vi "S2DS_Open dstp for external write (SubVI).vi"(8 "error in (no error)":errorcluster, 9 "Number identifier":i32, 10 "External Write instrument settings":T2={"Check for response?"=FALSE, "Pooling time out (ms)"=0, "Precision"=0.0, "IP"="localhost"}, 11 "Instrument parameters in":T1) -> (0 "error out":errorcluster, 1 "Read port list":string[](array[string]), 2 "Write port list":string[](array[string]), 3 "Instrument parameters out":T1)   [LabVIEW 2025]
uses:
  TYPE DEFS/S2DS_External write instrument settings.ctl
  TYPE DEFS/S2DS_Instrument parameters.ctl
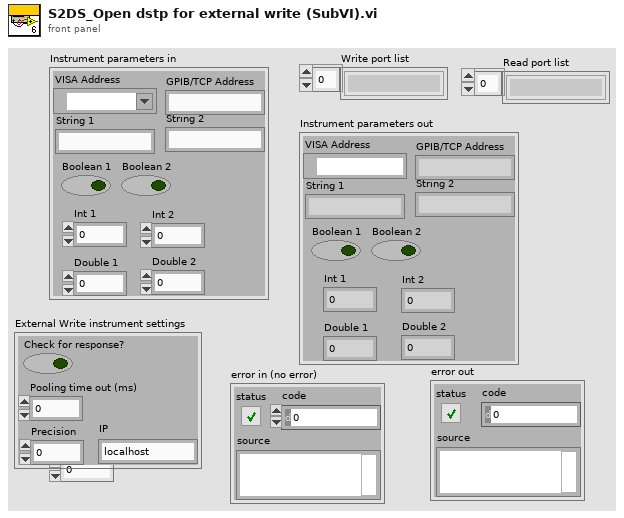
[diagram p1: front panel]
types:
  T1 = typedef "S2DS_Instrument parameters.ctl" = cluster{"VISA Address":refnum<visa-resource-name>, "GPIB/TCP Address":string, "String 1":string, "String 2":string, "Boolean 1":bool, "Boolean 2":bool, "Int 1":i32, "Int 2":i32, "Double 1":dbl, "Double 2":dbl}
  T2 = typedef "S2DS_External write instrument settings.ctl" = cluster{"Check for response?":bool, "Pooling time out (ms)":i32, "Precision":dbl, "IP":string}
  T3 = enum16{"Read", "Write", "ReadWrite", "BufferedRead", "BufferedReadWrite"}
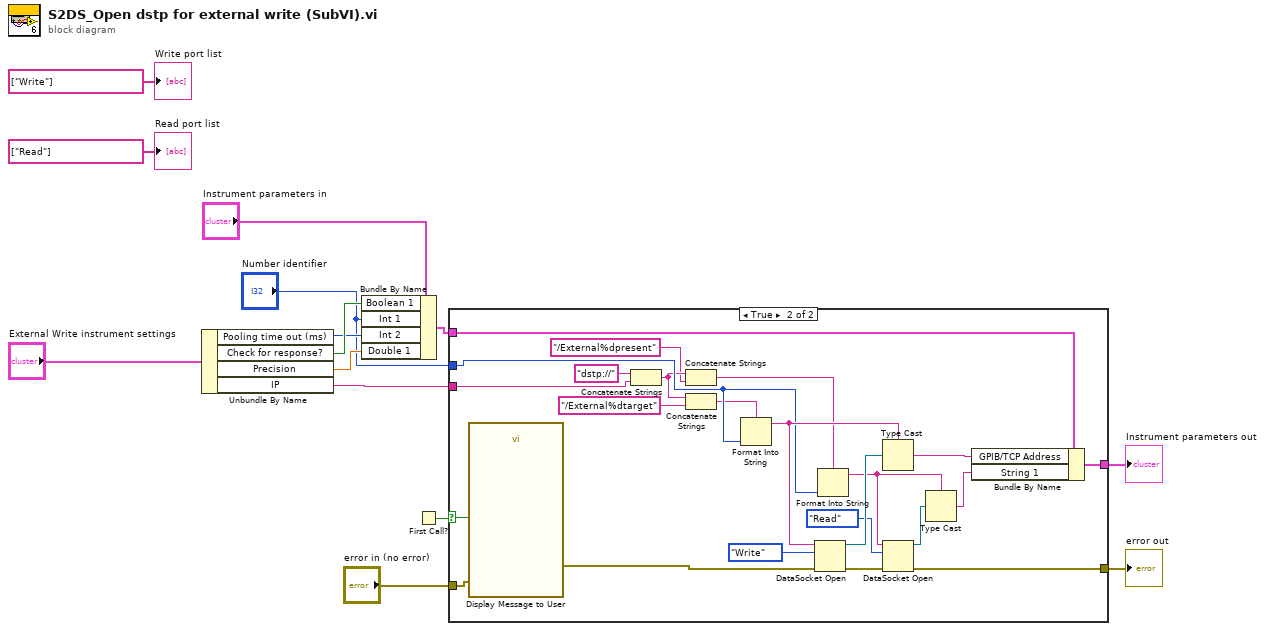
[diagram p0: block diagram]
diagram:
  n1 = Unbundle By Name("External Write instrument settings") -> ("Pooling time out (ms)"=w11:i32, "Check for response?"=w14:bool, "Precision"=w10:dbl, "IP"=w1:string)
  n2 = Bundle By Name(cluster="Instrument parameters in", "Boolean 1"=w14, "Int 1"="Number identifier", "Int 2"=w11, "Double 1"=w10) -> (w4:T1)
  n3 = First Call?() -> (First Call?: T/F=w9:bool)
  n4 = case shown="True" w9 {
    selector: w9 -> [_ w39]
    tunnel: [w16 w26] -> w7
    tunnel: "error in (no error)" -> [w16 w37]
    tunnel: w4 -> [w15 w36]
    tunnel: [w15 w35] -> w3
    tunnel: "Number identifier" -> [_ w30]
    tunnel: w1 -> [_ w22]
    frame False {
    }
    frame True {
      n5 = call "Display Message to User"("error in (no error)"=w37, "Enable"=w39) -> ("error out"=w38:errorcluster)  [unwired: 8 in, 1 out]
      n6 = Concatenate Strings("dstp://" ("string"), w22) -> (w21:string)
      n7 = Concatenate Strings(w21, "/External%dpresent" ("Write Location")) -> (w17:string)
      n8 = Concatenate Strings(w21, "/External%dtarget" ("Write Location")) -> (w19:string)
      n9 = Format Into String(format string=w19, w30) -> (resulting string=w33:string)  [unwired: 2 in, 1 out]
      n10 = DataSocket Open(8:w38, 10:T3."Write" ("mode"), 11:w33) -> (0:w27:errorcluster, 3:w34:refnum<k13>)  [unwired: 1 in]
      n11 = Format Into String(format string=w17, w30) -> (resulting string=w24:string)  [unwired: 2 in, 1 out]
      n12 = Type Cast(type=w33, x=w34) -> (*(type *) &x=w31:string)
      n13 = DataSocket Open(8:w27, 10:T3."Read" ("mode"), 11:w24) -> (0:w26:errorcluster, 3:w28:refnum<k13>)  [unwired: 1 in]
      n14 = Type Cast(type=w24, x=w28) -> (*(type *) &x=w25:string)
      n15 = Bundle By Name(cluster=w36, "GPIB/TCP Address"=w31, "String 1"=w25) -> (w35:T1)
    }
  }
  "Instrument parameters out" <- w3
  "error out" <- w7
  "Write port list" <- string[] ["Write"]
  "Read port list" <- string[] ["Read"]
